vi "BRig_dataBlock_c_nTrial_NFE.vi"() -> (2 "output_c_nTrial_NFE":i32)   [LabVIEW 2014]
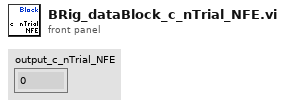
[diagram p1: front panel]
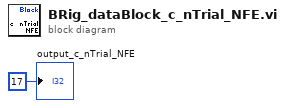
[diagram p0: block diagram]
diagram:
  "output_c_nTrial_NFE" <- 17 ("output_iBlock")
